vi "INIT.vi"(8 "error in (no error)":errorcluster, 11 "DelayLineSimulation in":refnum<class "DelayLineEmulate.lvclass">) -> (0 "error out":errorcluster, 3 "DelayLineSimulation out":refnum<class "DelayLineEmulate.lvclass">)   [LabVIEW 2015, in "DelayLineEmulate.lvclass"]
uses:
  DelayLineEmulate.lvclass
  GeneralFunctionality/GeneralFunctionality.lvclass/GeneralFunctionality.ctl
  dependecies/ControlsVIs/Clusters-def/SERVER-Commands.ctl
  dependecies/ControlsVIs/Clusters-def/Message types.ctl
  Control/Control-Server/Control-Server.lvclass
  Message/Message.lvclass
  GeneralFunctionality/GeneralFunctionality.lvclass
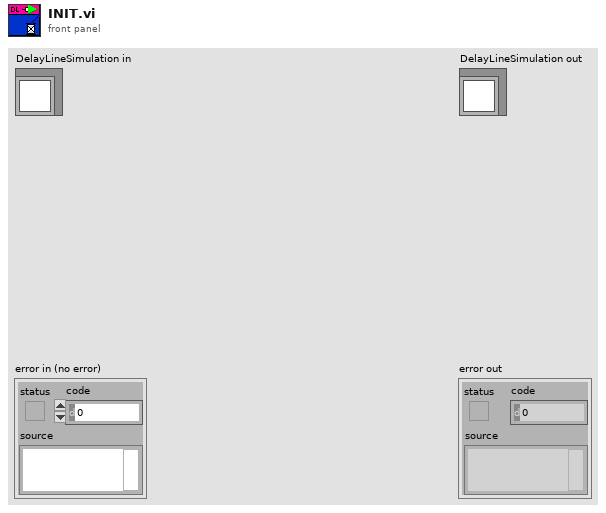
[diagram p1: front panel]
types:
  T1 = typedef "Message types.ctl" = string
  T2 = typedef "Control-Server.lvclass/SERVER-Commands.ctl" = string
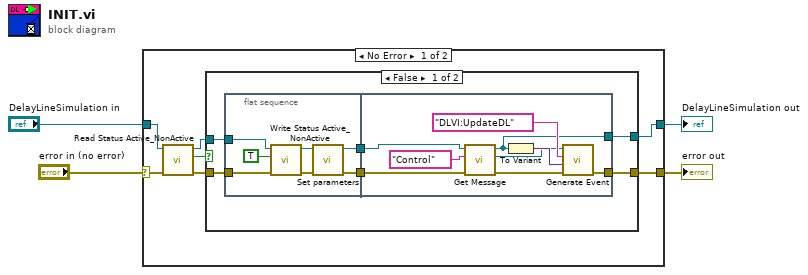
[diagram p0: block diagram]
diagram:
  n1 = case shown="No Error" "error in (no error)" {
    selector: "error in (no error)" -> [w8 w36]
    tunnel: "DelayLineSimulation in" -> [w9 w37]
    tunnel: [w11 w37] -> w1
    tunnel: [w10 w36] -> w2
    frame No Error {
      n2 = call "Read Status Active_NonActive.vi"("error in (no error)"=w8, "GeneralFunctionality in"=w9) -> ("error out"=w5:errorcluster, "Status Active/NonActive"=w7:bool, "GeneralFunctionality out"=w6:refnum<class "DelayLineEmulate.lvclass">)  [unwired: 7 in]
      n3 = case shown="False" w7 {
        tunnel: [w13 w35] -> w11
        tunnel: [w15 w34] -> w10
        tunnel: w6 -> [w17 w35]
        tunnel: w5 -> [w16 w34]
        frame False {
          n4 = flat-sequence {
            tunnel: w17 -> [w24]
            tunnel: w16 -> [w22]
            tunnel: [w20] -> w14
            tunnel: [w19] -> w12
            tunnel: w14 -> [w31]
            tunnel: [w29] -> w15
            tunnel: [w26] -> w13
            tunnel: w12 -> [w27]
            frame #0 {
              n5 = call "Write Status Active_NonActive.vi"("error in (no error)"=w22, "Status Active/NonActive"=TRUE, "GeneralFunctionality in"=w24) -> ("error out"=w21:errorcluster, "GeneralFunctionality out"=w18:refnum<class "DelayLineEmulate.lvclass">)  [unwired: 7 in]
              n6 = call-dynamic "Set parameters.vi"("error in (no error)"=w21, "DelayLineSimulation en entrée"=w18) -> ("error out"=w20:errorcluster, "DelayLineSimulation en sortie"=w19:refnum<class "DelayLineEmulate.lvclass">)  [unwired: 8 in]
            }
            frame #1 {
              n7 = call "Get Message.vi"("error in (no error)"=w31, "Message type"=T1 "Control", "GeneralFunctionality en entrée"=w27) -> ("error out"=w30:errorcluster, "Message.lvclass"=w28:refnum<class "Message.lvclass">, "GeneralFunctionality en sortie"=w26:refnum<class "DelayLineEmulate.lvclass">)  [unwired: 6 in]
              n8 = To Variant(anything=w26) -> (Variant=w33:variant)
              n9 = call "Generate Event.vi"("error in (no error)"=w30, "Data"=w33, "Command"=T2 "DLVI:UpdateDL", "Message en entrée"=w28) -> ("error out"=w29:errorcluster)  [unwired: 6 in, 1 out]
            }
          }
        }
        frame True {
        }
      }
    }
    frame Error {
    }
  }
  "error out" <- w2
  "DelayLineSimulation out" <- w1
